vi "Extension Control.vi"(0 "Pivot Stick":dbl, 1 "Is arm pivoting down?":bool, 2 "Extension Trigger":dbl, 3 "Retraction Trigger":dbl, 4 "Wrist Stick":dbl, 5 "Extention TPI":dbl, 6 "Pivot Position":dbl, 7 "Is wrist pivoting down?":bool, 8 "Pivot TPR":dbl, 9 "Current highest point of arm":dbl, 10 "Extention Position":dbl, 12 "Extending and above max height?":bool) -> ()   [LabVIEW 2014]
uses:
  Robot Global Data.vi
panel:
  out "Extention Output":dbl
  in  "Wrist TPR":dbl
  in  "Wrist Position":dbl
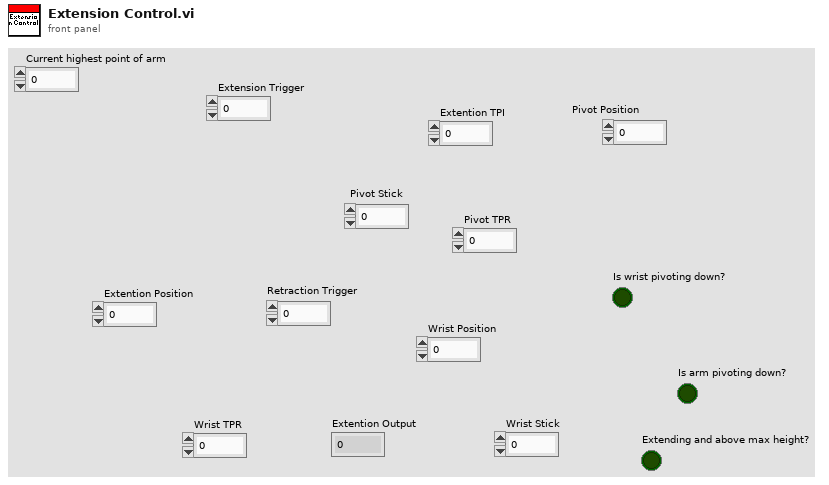
[diagram p1: front panel]
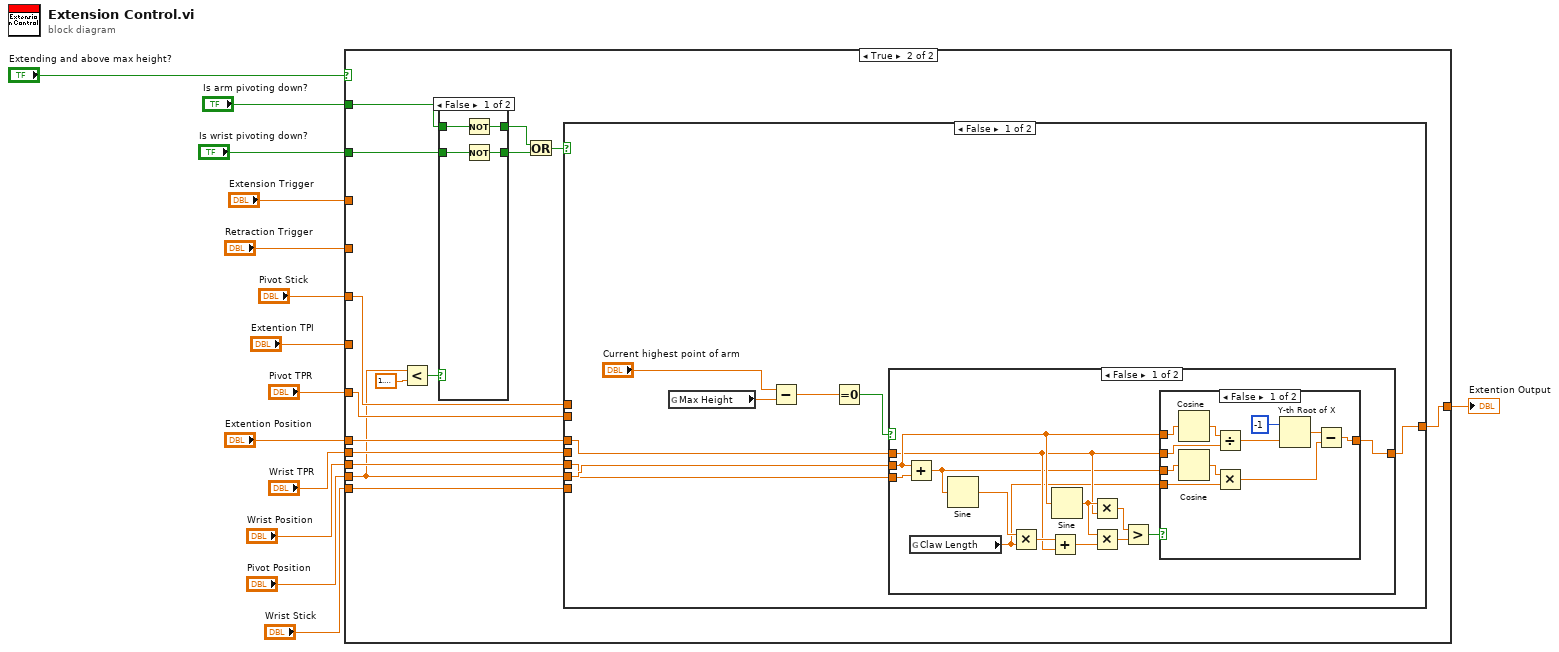
[diagram p0: block diagram]
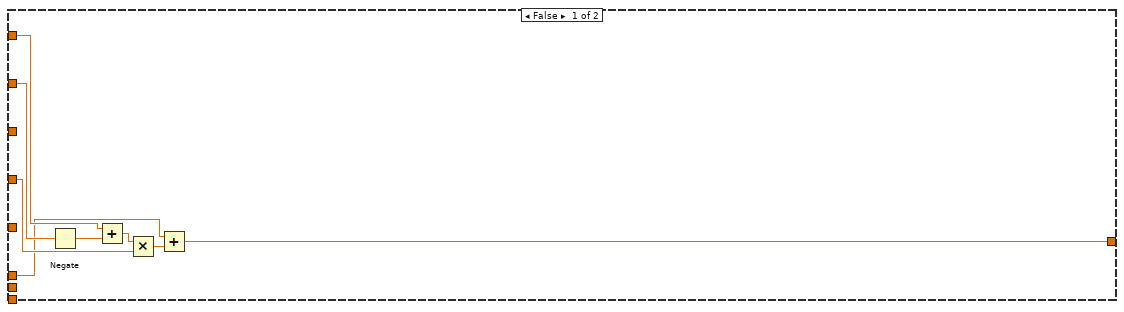
[diagram p2: hidden frame]
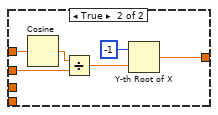
[diagram p4: hidden frame]
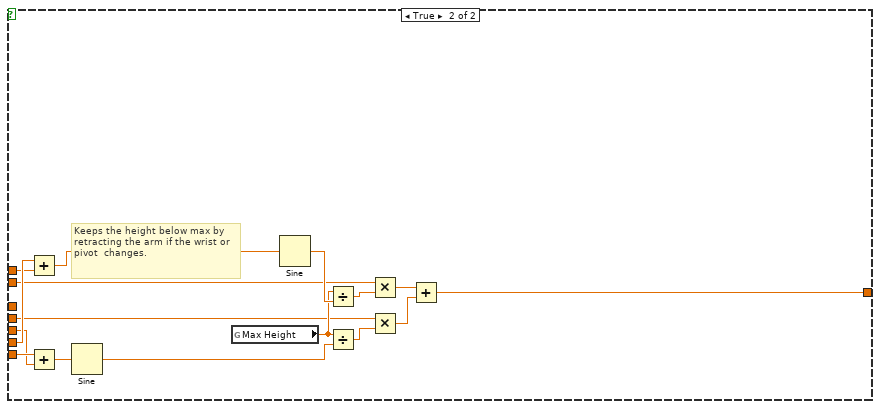
[diagram p6: hidden frame]
diagram:
  n1 = case shown="True" "Extending and above max height?" {
    tunnel: "Extension Trigger" -> [w22 _]
    tunnel: "Retraction Trigger" -> [w21 _]
    tunnel: "Extention TPI" -> [w17 _]
    tunnel: [w16 w31] -> w1
    tunnel: "Is arm pivoting down?" -> [_ w28]
    tunnel: "Pivot Stick" -> [_ w36]
    tunnel: "Wrist Stick" -> [_ w35]
    tunnel: "Pivot Position" -> [_ w27]
    tunnel: "Wrist Position" -> [_ w34]
    tunnel: "Wrist TPR" -> [_ w33]
    tunnel: "Pivot TPR" -> [_ w32]
    tunnel: "Extention Position" -> [w15 w30]
    tunnel: "Is wrist pivoting down?" -> [_ w24]
    frame False {
      n2 = Negate(x=w21) -> (-x=w20:dbl)
      n3 = Add(x=w22, y=w20) -> (x+y=w19:dbl)
      n4 = Multiply(x=w19, y=w17) -> (x*y=w18:dbl)
      n5 = Add(x=w15, y=w18) -> (x+y=w16:dbl)
    }
    frame True {
      n6 = Less?(x=w27, y=1.5707963267948966) -> (x < y?=w26:bool)
      n7 = case shown="False" w26 {
        tunnel: [w41 w43] -> w29
        tunnel: w28 -> [w40 w43]
        tunnel: w24 -> [w39 w42]
        tunnel: [w38 w42] -> w23
        frame False {
          n8 = Not(x=w40) -> (.not. x?=w41:bool)
          n9 = Not(x=w39) -> (.not. x?=w38:bool)
        }
        frame True {
        }
      }
      n10 = Or(x=w29, y=w23) -> (x .or. y?=w37:bool)
      n11 = case shown="False" w37 {
        tunnel: w36 -> [_ w83]
        tunnel: w35 -> [_ w90]
        tunnel: w27 -> [w46 w98]
        tunnel: w34 -> [w45 w89]
        tunnel: w33 -> [_ w88]
        tunnel: w32 -> [_ w87]
        tunnel: [w44 w84] -> w31
        tunnel: w30 -> [w51 _]
        frame False {
          n12 = global read "Robot Global Data.vi" "Max Height"() -> (w50:dbl)
          n13 = Subtract(x="Current highest point of arm", y=w50) -> (x-y=w48:dbl)
          n14 = Equal To 0?(x=w48) -> (x = 0?=w47:bool)
          n15 = case shown="False" w47 {
            tunnel: [w55 w82] -> w44
            tunnel: w51 -> [w56 w82]
            tunnel: w46 -> [w57 _]
            tunnel: w45 -> [w54 _]
            frame False {
              n16 = Add(x=w57, y=w54) -> (x+y=w52:dbl)
              n17 = global read "Robot Global Data.vi" "Claw Length"() -> (w53:dbl)
              n18 = Sine(x=w52) -> (sin(x)=w61:dbl)
              n19 = Multiply(x=w61, y=w53) -> (x*y=w63:dbl)
              n20 = Add(x=w63, y=w56) -> (x+y=w62:dbl)
              n21 = Sine(x=w57) -> (sin(x)=w64:dbl)
              n22 = Multiply(x=w64, y=w56) -> (x*y=w60:dbl)
              n23 = Multiply(x=w64, y=w62) -> (x*y=w59:dbl)
              n24 = Greater?(x=w60, y=w59) -> (0:w58:bool)
              n25 = case shown="False" w58 {
                tunnel: w57 -> [w71 w81]
                tunnel: w56 -> [w72 w80]
                tunnel: [w66 w76] -> w55
                tunnel: w53 -> [w69 _]
                tunnel: w52 -> [w65 _]
                frame False {
                  n26 = Cosine(x=w71) -> (cos(x)=w75:dbl)
                  n27 = Cosine(x=w65) -> (cos(x)=w70:dbl)
                  n28 = Divide(x=w75, y=w72) -> (x/y=w73:dbl)
                  n29 = Multiply(x=w70, y=w69) -> (x*y=w67:dbl)
                  n30 = Y-th Root of X(1:w73, 2:-1) -> (0:w68:dbl)
                  n31 = Subtract(x=w68, y=w67) -> (x-y=w66:dbl)
                }
                frame True {
                  n32 = Cosine(x=w81) -> (cos(x)=w79:dbl)
                  n33 = Divide(x=w79, y=w80) -> (x/y=w77:dbl)
                  n34 = Y-th Root of X(1:w77, 2:-1) -> (0:w76:dbl)
                }
              }
            }
            frame True {
            }
          }
        }
        frame True {
          # "Keeps the height below max by retracting the arm if the wrist or pivot  changes."
          n35 = Add(x=w98, y=w83) -> (x+y=w97:dbl)
          n36 = Add(x=w90, y=w89) -> (x+y=w94:dbl)
          n37 = Sine(x=w94) -> (sin(x)=w93:dbl)
          n38 = global read "Robot Global Data.vi" "Max Height"() -> (w91:dbl)
          n39 = Sine(x=w97) -> (sin(x)=w96:dbl)
          n40 = Divide(x=w91, y=w96) -> (x/y=w95:dbl)
          n41 = Divide(x=w91, y=w93) -> (x/y=w92:dbl)
          n42 = Multiply(x=w87, y=w95) -> (x*y=w86:dbl)
          n43 = Multiply(x=w88, y=w92) -> (x*y=w85:dbl)
          n44 = Add(x=w86, y=w85) -> (x+y=w84:dbl)
        }
      }
    }
  }
  "Extention Output" <- w1
